vi "Get_Set_Statistics.vi"(1 "Value in":T1={"Thresh_Count_MAS"={"Sing_Ch1_low"=0, "Sing_Ch1_high"=0, "Sing_Ch2_low"=0, "Sing_Ch2_high"=0, "Total_Ch1_low"=0, "Total_Ch1_high"=0, "Total_Ch2_low"=0, "Total_Ch2_high"=0, "Av_Ch1_low"=0.0, "Av_Ch1_high"=0.0, "Av_Ch2_low"=0.0, "Av_Ch2_high"=0.0}, "Thresh_Count_SLV"={"Sing_Ch1_low"=0, "Sing_Ch1_high"=0, "Sing_Ch2_low"=0, "Sing_Ch2_high"=0, "Total_Ch1_low"=0, "Total_Ch1_high"=0, "Total_Ch2_low"=0, "Total_Ch2_high"=0, "Av_Ch1_low"=0.0, "Av_Ch1_high"=0.0, "Av_Ch2_low"=0.0, "Av_Ch2_high"=0.0}, "Count"=FALSE, "Time_to_count"=60, "Time"=0, "Time_to_count_ref"=refnum, "Counting?"=FALSE, "Baseline_MAS_Ch1"=0, "Baseline_MAS_Ch2"=0, "Baseline_SLV_Ch1"=0, "Baseline_SLV_Ch2"=0, "Basel_Err_MAS_Ch1"=0, "Basel_Err_MAS_Ch2"=0, "Basel_Err_SLV_Ch1"=0, "Basel_Err_SLV_Ch2"=0, "Peaks_Overshoot"=0.0, "Height_Overshoot"=0.0, "Integrals_Overshoot"=0.0, "Last_event"=0.0, "Total_Trigger"=0, "Av_Trigger"=0.0, "Number of peaks"={"t0"=0, "dt"=0, "Histogram"=[]}, "Pulse height"={"t0"=0, "dt"=0, "Histogram"=[]}, "Integral"={"t0"=0, "dt"=0, "Histogram"=[]}, "Number of peaks Entries"=0, "Number of peaks Overshoots"=0, "Pulse height  Entries"=0, "Pulse height Overshoots"=0, "Integral Entries"=0, "Integral Overshoots"=0, "Last trigger Stack"=refnum} {"Av_Trigger" format="%#_3g"; "Last_event" format="%#_3g"; "Integrals_Overshoot" format="%#_2f"; "Height_Overshoot" format="%#_2f"; "Peaks_Overshoot" format="%#_2f"; "Thresh_Count_SLV"."Av_Ch2_high" format="%#.2g"; "Thresh_Count_SLV"."Av_Ch2_low" format="%#.2g"; "Thresh_Count_SLV"."Av_Ch1_high" format="%#.2g"; "Thresh_Count_SLV"."Av_Ch1_low" format="%#.2g"; "Thresh_Count_MAS"."Av_Ch2_high" format="%#.2g"; "Thresh_Count_MAS"."Av_Ch2_low" format="%#.2g"; "Thresh_Count_MAS"."Av_Ch1_high" format="%#.2g"; "Thresh_Count_MAS"."Av_Ch1_low" format="%#.2g"}, 2 "Page Statistics in":refnum<vi>, 3 "Status/Errors in":refnum<vi>, 4 "Get/Set":T3) -> (8 "Value out":T1={"Thresh_Count_MAS"={"Sing_Ch1_low"=0, "Sing_Ch1_high"=0, "Sing_Ch2_low"=0, "Sing_Ch2_high"=0, "Total_Ch1_low"=0, "Total_Ch1_high"=0, "Total_Ch2_low"=0, "Total_Ch2_high"=0, "Av_Ch1_low"=0.0, "Av_Ch1_high"=0.0, "Av_Ch2_low"=0.0, "Av_Ch2_high"=0.0}, "Thresh_Count_SLV"={"Sing_Ch1_low"=0, "Sing_Ch1_high"=0, "Sing_Ch2_low"=0, "Sing_Ch2_high"=0, "Total_Ch1_low"=0, "Total_Ch1_high"=0, "Total_Ch2_low"=0, "Total_Ch2_high"=0, "Av_Ch1_low"=0.0, "Av_Ch1_high"=0.0, "Av_Ch2_low"=0.0, "Av_Ch2_high"=0.0}, "Count"=FALSE, "Time_to_count"=60, "Time"=0, "Time_to_count_ref"=refnum, "Counting?"=FALSE, "Baseline_MAS_Ch1"=0, "Baseline_MAS_Ch2"=0, "Baseline_SLV_Ch1"=0, "Baseline_SLV_Ch2"=0, "Basel_Err_MAS_Ch1"=0, "Basel_Err_MAS_Ch2"=0, "Basel_Err_SLV_Ch1"=0, "Basel_Err_SLV_Ch2"=0, "Peaks_Overshoot"=0.0, "Height_Overshoot"=0.0, "Integrals_Overshoot"=0.0, "Last_event"=0.0, "Total_Trigger"=0, "Av_Trigger"=0.0, "Number of peaks"={"t0"=0, "dt"=0, "Histogram"=[]}, "Pulse height"={"t0"=0, "dt"=0, "Histogram"=[]}, "Integral"={"t0"=0, "dt"=0, "Histogram"=[]}, "Number of peaks Entries"=0, "Number of peaks Overshoots"=0, "Pulse height  Entries"=0, "Pulse height Overshoots"=0, "Integral Entries"=0, "Integral Overshoots"=0, "Last trigger Stack"=refnum} {"Av_Trigger" format="%#_3g"; "Last_event" format="%#_3g"; "Integrals_Overshoot" format="%#_2f"; "Height_Overshoot" format="%#_2f"; "Peaks_Overshoot" format="%#_2f"; "Thresh_Count_SLV"."Av_Ch2_high" format="%#.2g"; "Thresh_Count_SLV"."Av_Ch2_low" format="%#.2g"; "Thresh_Count_SLV"."Av_Ch1_high" format="%#.2g"; "Thresh_Count_SLV"."Av_Ch1_low" format="%#.2g"; "Thresh_Count_MAS"."Av_Ch2_high" format="%#.2g"; "Thresh_Count_MAS"."Av_Ch2_low" format="%#.2g"; "Thresh_Count_MAS"."Av_Ch1_high" format="%#.2g"; "Thresh_Count_MAS"."Av_Ch1_low" format="%#.2g"}, 9 "Page Statistics out":refnum<vi>, 10 "Status/Errors out":refnum<vi>)   [LabVIEW 2013]
uses:
  Controls/Get_Set_Statistics_Options.ctl
  Controls/TabPage_Statistics.ctl
  Controls/Page_Thresholds.ctl
panel:
  # "Number of peaks"
  # "Pulse height"
  # "Integral"
  # "Running average (Hz)"
  # "Counts"
  # "M A S T E R   D E V I C E"
  # "Trigger rate"
  # "S L A V E   D E V I C E"
  # "# errors in baseline"
  # "Baselines (ADC counts)"
  # "Singles"
  # "Last second"
  # "Total"
  # "Average per second"
  # "Channel 1 - low"
  # "Channel 1 - high"
  # "Channel 2 - low"
  # "Channel 2 - high"
  # "Singles"
  # "Last second"
  # "Total"
  # "Average per second"
  # "Channel 1 - low"
  # "Channel 1 - high"
  # "Channel 2 - low"
  # "Channel 2 - high"
  # "Number of peaks"
  # "Pulse height"
  # "Integral"
  # "Running average (Hz)"
  # "Counts"
  # "M A S T E R   D E V I C E"
  # "Trigger rate"
  # "S L A V E   D E V I C E"
  # "# errors in baseline"
  # "Baselines (ADC counts)"
  # "Singles"
  # "Last second"
  # "Total"
  # "Average per second"
  # "Channel 1 - low"
  # "Channel 1 - high"
  # "Channel 2 - low"
  # "Channel 2 - high"
  # "Singles"
  # "Last second"
  # "Total"
  # "Average per second"
  # "Channel 1 - low"
  # "Channel 1 - high"
  # "Channel 2 - low"
  # "Channel 2 - high"
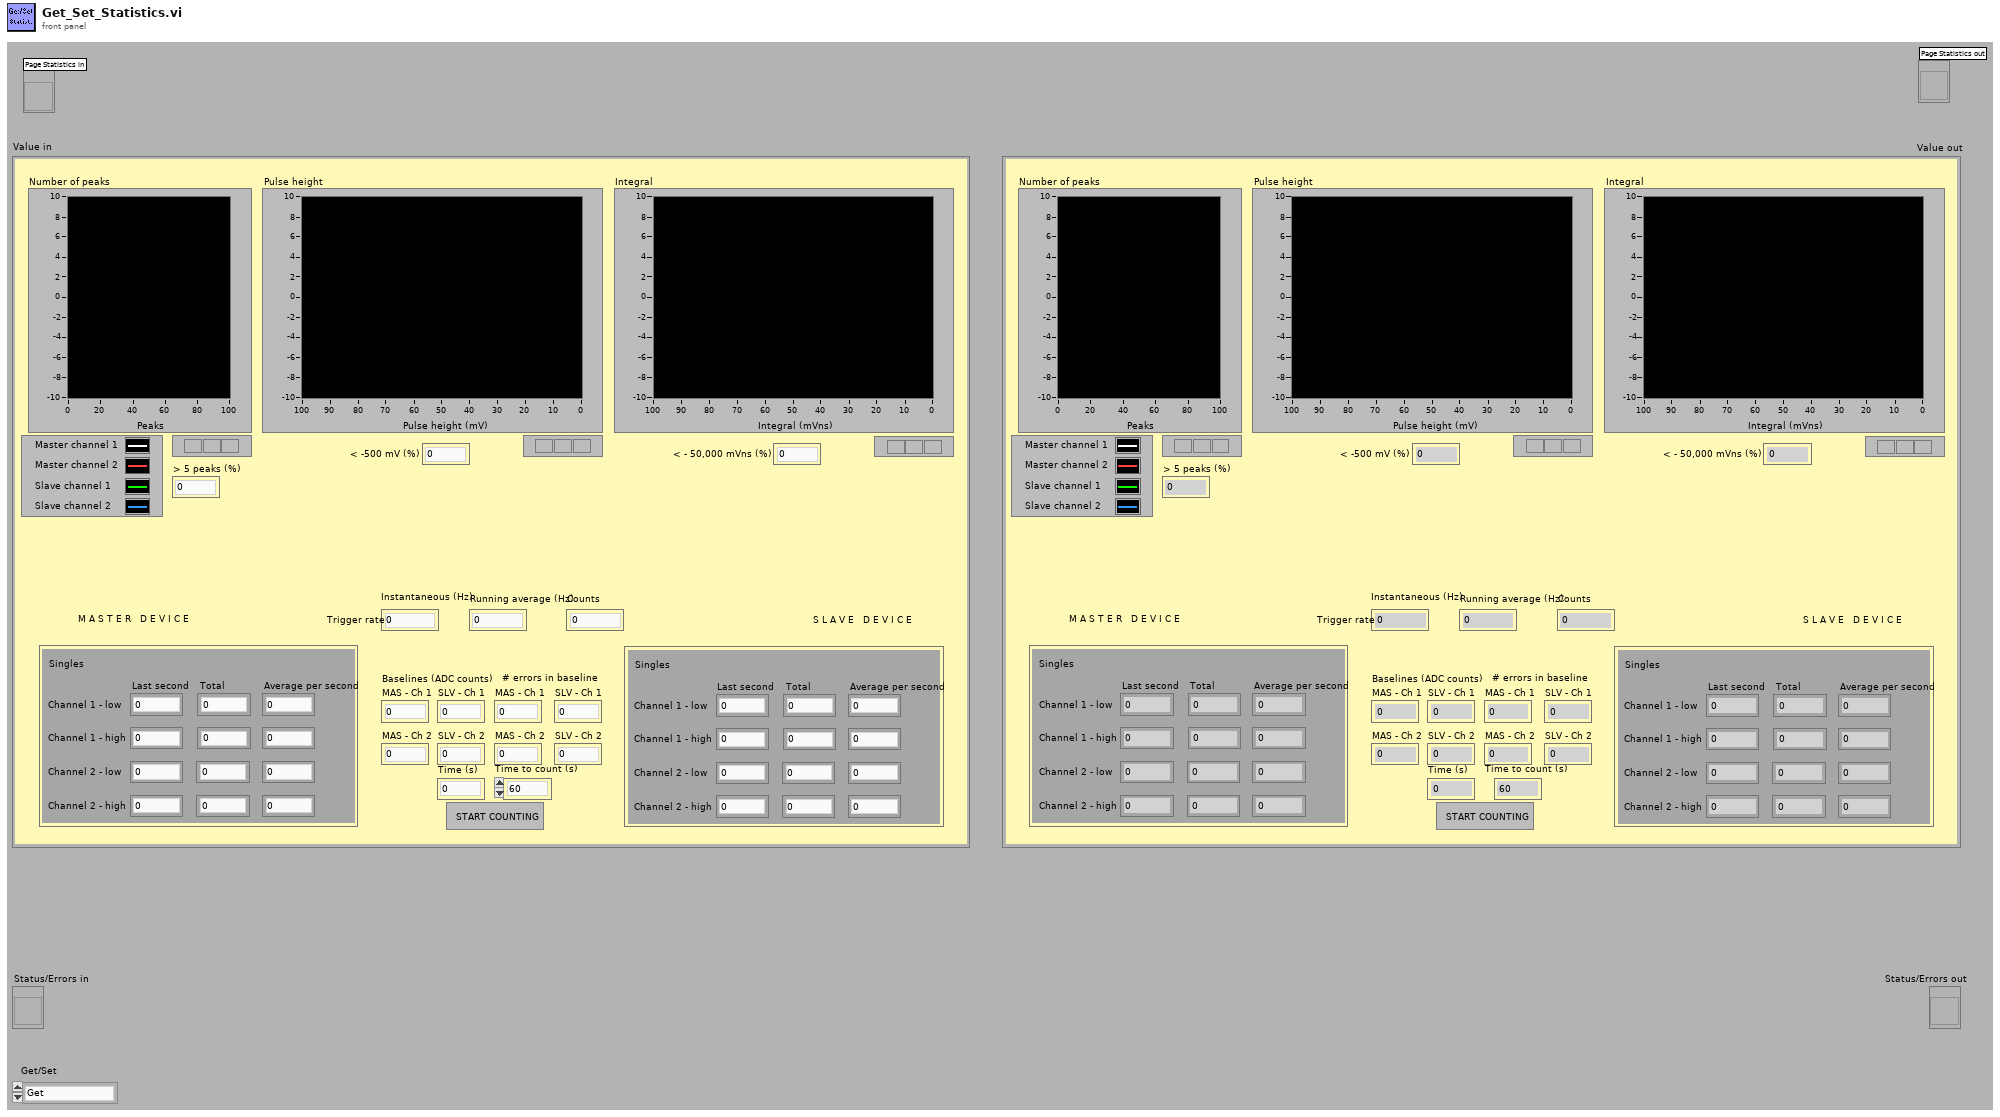
[diagram p1: front panel]
types:
  T1 = typedef "TabPage_Statistics.ctl" = cluster{"Thresh_Count_MAS":T2, "Thresh_Count_SLV":T2, "Count":bool, "Time_to_count":u32, "Time":u32, "Time_to_count_ref":refnum<vi>, "Counting?":bool, "Baseline_MAS_Ch1":i16, "Baseline_MAS_Ch2":i16, "Baseline_SLV_Ch1":i16, "Baseline_SLV_Ch2":i16, "Basel_Err_MAS_Ch1":u32, "Basel_Err_MAS_Ch2":u32, "Basel_Err_SLV_Ch1":u32, "Basel_Err_SLV_Ch2":u32, "Peaks_Overshoot":dbl, "Height_Overshoot":dbl, "Integrals_Overshoot":dbl, "Last_event":dbl, "Total_Trigger":u32, "Av_Trigger":dbl, "Number of peaks":cluster{"t0":i32, "dt":i32, "Histogram":i32[][]}, "Pulse height":cluster{"t0":i32, "dt":i32, "Histogram":i32[][]}, "Integral":cluster{"t0":i32, "dt":i32, "Histogram":i32[][]}, "Number of peaks Entries":u64, "Number of peaks Overshoots":u64, "Pulse height  Entries":u64, "Pulse height Overshoots":u64, "Integral Entries":u64, "Integral Overshoots":u64, "Last trigger Stack":refnum<vi>}
  T2 = typedef "Page_Thresholds.ctl" = cluster{"Sing_Ch1_low":u32, "Sing_Ch1_high":u32, "Sing_Ch2_low":u32, "Sing_Ch2_high":u32, "Total_Ch1_low":u32, "Total_Ch1_high":u32, "Total_Ch2_low":u32, "Total_Ch2_high":u32, "Av_Ch1_low":dbl, "Av_Ch1_high":dbl, "Av_Ch2_low":dbl, "Av_Ch2_high":dbl}
  T3 = typedef "Get_Set_Statistics_Options.ctl" = enum16{"Get", "Set singles", "Set events"}
  T4 = cluster{"Thresh_Count_MAS":T2, "Thresh_Count_SLV":T2, "Count":bool, "Time_to_count":u32, "Time":u32, "Time_to_count_ref":refnum<vi>, "Counting?":bool, "Baseline_MAS_Ch1":i16, "Baseline_MAS_Ch2":i16, "Baseline_SLV_Ch1":i16, "Baseline_SLV_Ch2":i16, "Basel_Err_MAS_Ch1":u32, "Basel_Err_MAS_Ch2":u32, "Basel_Err_SLV_Ch1":u32, "Basel_Err_SLV_Ch2":u32, "Peaks_Overshoot":dbl, "Height_Overshoot":dbl, "Integrals_Overshoot":dbl, "Last_event":dbl, "Total_Trigger":u32, "Av_Trigger":dbl, "Number of peaks":cluster{"t0":i32, "dt":i32, "Histogram":i32[][]}, "Pulse height":cluster{"t0":i32, "dt":i32, "Histogram":i32[][]}, "Integral":cluster{"t0":i32, "dt":i32, "Histogram":i32[][]}, "Number of peaks Entries":u64, "Number of peaks Overshoots":u64, "Pulse height  Entries":u64, "Pulse height Overshoots":u64, "Integral Entries":u64, "Integral Overshoots":u64, "Last trigger Stack":refnum<vi>}
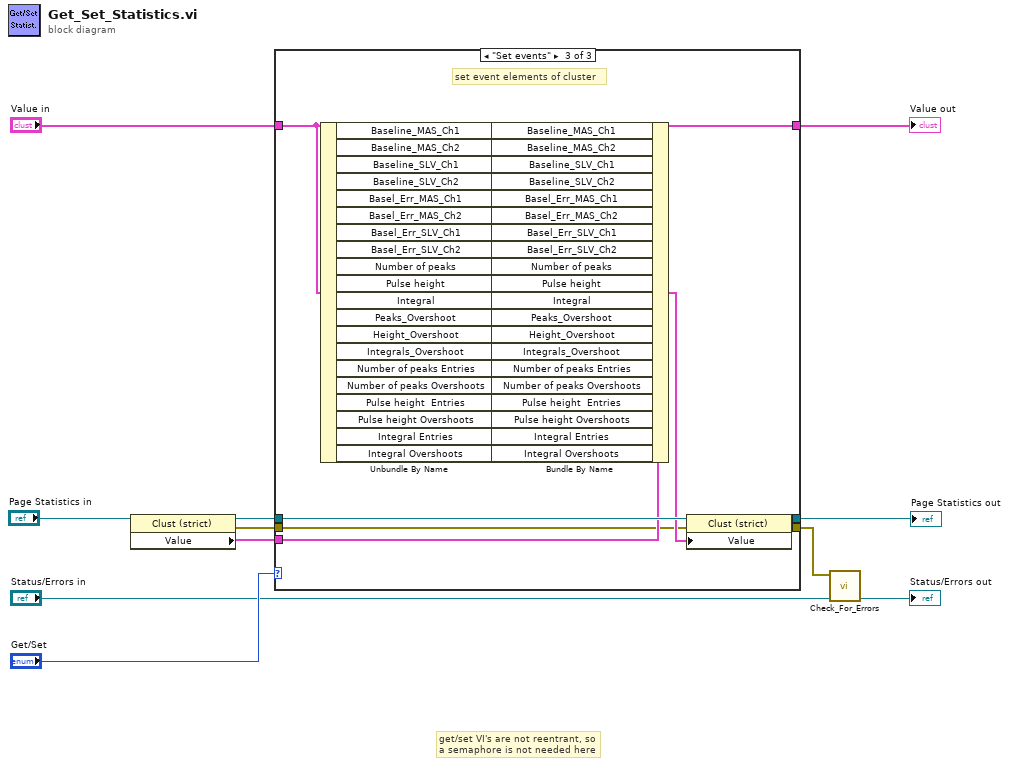
[diagram p0: block diagram]
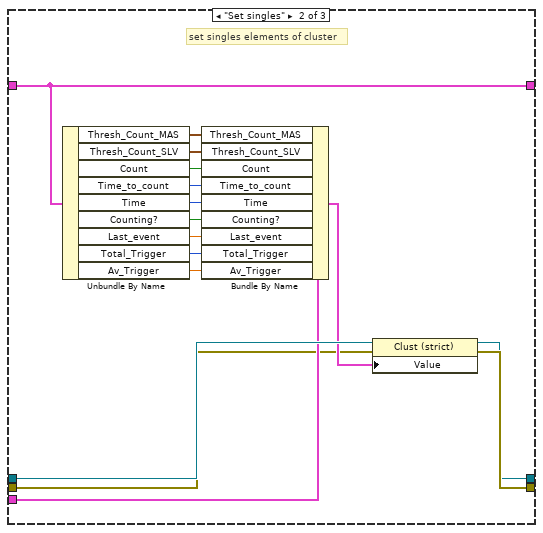
[diagram p3: hidden frame]
diagram:
  # "get/set VI's are not reentrant, so\na semaphore is not needed here"
  n1 = property class="Clust (strict)"(reference="Page Statistics in") -> (reference out=w6:refnum<vi>, error out=w4:errorcluster, "Value"=w5:T4)  [unwired: 1 in]
  n2 = case shown="\"Set events\"" "Get/Set" {
    tunnel: "Value in" -> [_ w26 w53]
    tunnel: w6 -> [w14 w30 w57]
    tunnel: [w14 w28 w55] -> w2
    tunnel: [w13 w29 w56] -> w9
    tunnel: [w12 w26 w53] -> w3
    tunnel: w5 -> [w12 w27 w54]
    tunnel: w4 -> [w13 w18 w40]
    frame "Get" {
      # "get cluster"
    }
    frame "Set singles" {
      # "set singles elements of cluster"
      n3 = Unbundle By Name(w26) -> ("Thresh_Count_MAS"=w25:T2, "Thresh_Count_SLV"=w24:T2, "Count"=w23:bool, "Time_to_count"=w22:u32, "Time"=w21:u32, "Counting?"=w20:bool, "Last_event"=w17:dbl, "Total_Trigger"=w16:u32, "Av_Trigger"=w15:dbl)
      n4 = Bundle By Name(cluster=w27, "Thresh_Count_MAS"=w25, "Thresh_Count_SLV"=w24, "Count"=w23, "Time_to_count"=w22, "Time"=w21, "Counting?"=w20, "Last_event"=w17, "Total_Trigger"=w16, "Av_Trigger"=w15) -> (w19:T4)
      n5 = property class="Clust (strict)"(reference=w30, error in=w18, "Value"=w19) -> (reference out=w28:refnum<vi>, error out=w29:errorcluster)
    }
    frame "Set events" {
      # "set event elements of cluster"
      n6 = Unbundle By Name(w53) -> ("Baseline_MAS_Ch1"=w52:i16, "Baseline_MAS_Ch2"=w51:i16, "Baseline_SLV_Ch1"=w50:i16, "Baseline_SLV_Ch2"=w49:i16, "Basel_Err_MAS_Ch1"=w48:u32, "Basel_Err_MAS_Ch2"=w47:u32, "Basel_Err_SLV_Ch1"=w46:u32, "Basel_Err_SLV_Ch2"=w45:u32, "Number of peaks"=w44:cluster{"t0":i32, "dt":i32, "Histogram":i32[][]}, "Pulse height"=w43:cluster{"t0":i32, "dt":i32, "Histogram":i32[][]}, "Integral"=w42:cluster{"t0":i32, "dt":i32, "Histogram":i32[][]}, "Peaks_Overshoot"=w39:dbl, "Height_Overshoot"=w38:dbl, "Integrals_Overshoot"=w37:dbl, "Number of peaks Entries"=w36:u64, "Number of peaks Overshoots"=w35:u64, "Pulse height  Entries"=w34:u64, "Pulse height Overshoots"=w33:u64, "Integral Entries"=w32:u64, "Integral Overshoots"=w31:u64)
      n7 = Bundle By Name(cluster=w54, "Baseline_MAS_Ch1"=w52, "Baseline_MAS_Ch2"=w51, "Baseline_SLV_Ch1"=w50, "Baseline_SLV_Ch2"=w49, "Basel_Err_MAS_Ch1"=w48, "Basel_Err_MAS_Ch2"=w47, "Basel_Err_SLV_Ch1"=w46, "Basel_Err_SLV_Ch2"=w45, "Number of peaks"=w44, "Pulse height"=w43, "Integral"=w42, "Peaks_Overshoot"=w39, "Height_Overshoot"=w38, "Integrals_Overshoot"=w37, "Number of peaks Entries"=w36, "Number of peaks Overshoots"=w35, "Pulse height  Entries"=w34, "Pulse height Overshoots"=w33, "Integral Entries"=w32, "Integral Overshoots"=w31) -> (w41:T4)
      n8 = property class="Clust (strict)"(reference=w57, error in=w40, "Value"=w41) -> (reference out=w55:refnum<vi>, error out=w56:errorcluster)
    }
  }
  "Value out" <- w3
  "Page Statistics out" <- w2
  n9 = call "Check_For_Errors.vi"("Status/Errors in"="Status/Errors in", "error in"=w9) -> ("Status/Errors out"=→"Status/Errors out":refnum<vi>)  [unwired: 9 out]
